vi "FRIC_navX_Get_NextState_ProcessLoop.vi"(11 "I2C Process Loop TypeDef (in)":T1={"State Array"=[enum."INI", enum."Open"], "error"={"status"=FALSE, "code"=0, "source"=""}, "FPGA Cluster"={"Last Valid FPGA Time"=0.0, "Error Count"=0, "Initialized"=FALSE}, "Device Info"={"Interface"={"Protocol"=enum."SERIAL", "Update Rate (4Hz-100Hz)"=4, "navX Open TypeDef"=variant}, "Notify Packet"=refnum, "Loop VI Refnum"=refnum, "Ready to Close Occurrence Refnum"=refnum}, "I2CDevRef"={"DevStatus"={"status"=FALSE, "code"=0, "source"=""}, "Device Address"=0, "Handle"=0, "I2C Bus"=enum."Invalid"}, "Registry"=[], "Command Array"=[214, 32], "Connected?"=FALSE, "navX Device Memory Size"=85, "notification"={"navX Action"=enum."None", "Data"=variant}, "Memory Size Set"=FALSE, "SPIDevRef"={"DevStatus"={"status"=FALSE, "code"=0, "source"=""}, "Handle"=0, "SPI Bus"=enum."SPI On-Board, CS0"}, "navX Serial Open"={"Stream Type"=enum."YRPH", "Serial Port"=enum."Onboard RS-232"}, "SerialPortRef"={"DevStatus"={"status"=FALSE, "code"=0, "source"=""}, "Serial Port Name"=""}, "Serial Read Buffer"="", "Serial Write Buffer"=[], "Device Number"=enum."Dev0", "navX SPI Open"={"SPI Bus"=enum."SPI MXP", "Clock Rate (Hz)"=500000.0}, "Loop dt"=0, "current time"=timestamp(0 s since 1904-01-01), "Loop Time"=0} {"navX Device Memory Size" format="%x"; "Command Array" items=["UNDEFINED"=0, "NAVX_INTEGRATION_CTL_RESET_VEL_X"=1, "NAVX_INTEGRATION_CTL_RESET_VEL_Y"=2, "NAVX_INTEGRATION_CTL_RESET_VEL_Z"=4, "NAVX_INTEGRATION_CTL_RESET_DISP_X"=8, "NAVX_INTEGRATION_CTL_RESET_DISP_Y"=16, "NAVX_INTEGRATION_CTL_RESET_DISP_Z"=32, "NAVX_INTEGRATION_CTL_RESET_YAW"=128]; "I2CDevRef"."Device Address" format="%.0x"; "Device Info"."Interface"."Update Rate (4Hz-100Hz)" min=4 max=60 step=1}) -> (3 "I2C Process Loop TypeDef (out)":T1={"State Array"=[enum."INI", enum."Open"], "error"={"status"=FALSE, "code"=0, "source"=""}, "FPGA Cluster"={"Last Valid FPGA Time"=0.0, "Error Count"=0, "Initialized"=FALSE}, "Device Info"={"Interface"={"Protocol"=enum."SERIAL", "Update Rate (4Hz-100Hz)"=4, "navX Open TypeDef"=variant}, "Notify Packet"=refnum, "Loop VI Refnum"=refnum, "Ready to Close Occurrence Refnum"=refnum}, "I2CDevRef"={"DevStatus"={"status"=FALSE, "code"=0, "source"=""}, "Device Address"=0, "Handle"=0, "I2C Bus"=enum."Invalid"}, "Registry"=[], "Command Array"=[214, 32], "Connected?"=FALSE, "navX Device Memory Size"=85, "notification"={"navX Action"=enum."None", "Data"=variant}, "Memory Size Set"=FALSE, "SPIDevRef"={"DevStatus"={"status"=FALSE, "code"=0, "source"=""}, "Handle"=0, "SPI Bus"=enum."SPI On-Board, CS0"}, "navX Serial Open"={"Stream Type"=enum."YRPH", "Serial Port"=enum."Onboard RS-232"}, "SerialPortRef"={"DevStatus"={"status"=FALSE, "code"=0, "source"=""}, "Serial Port Name"=""}, "Serial Read Buffer"="", "Serial Write Buffer"=[], "Device Number"=enum."Dev0", "navX SPI Open"={"SPI Bus"=enum."SPI MXP", "Clock Rate (Hz)"=500000.0}, "Loop dt"=0, "current time"=timestamp(0 s since 1904-01-01), "Loop Time"=0} {"navX Device Memory Size" format="%x"; "Command Array" items=["UNDEFINED"=0, "NAVX_INTEGRATION_CTL_RESET_VEL_X"=1, "NAVX_INTEGRATION_CTL_RESET_VEL_Y"=2, "NAVX_INTEGRATION_CTL_RESET_VEL_Z"=4, "NAVX_INTEGRATION_CTL_RESET_DISP_X"=8, "NAVX_INTEGRATION_CTL_RESET_DISP_Y"=16, "NAVX_INTEGRATION_CTL_RESET_DISP_Z"=32, "NAVX_INTEGRATION_CTL_RESET_YAW"=128]; "I2CDevRef"."Device Address" format="%.0x"; "Device Info"."Interface"."Update Rate (4Hz-100Hz)" min=4 max=60 step=1}, 5 "Current State":T2)   [LabVIEW 2016]
uses:
  TypeDefs/FRIC_navX_I2C Process Loop TypeDef.ctl
  TypeDefs/FRIC_navX_ProcessingLoopStatesTypeDef_I2C.ctl
  TypeDefs/Z900_navX_DeviceTypeDef.ctl
  TypeDefs/Z900_navX_ProtocolTypeDef.ctl
  TypeDefs/Z900_navX_NotifyPacketTypeDef.ctl
  TypeDefs/Z900_navX_ActionTypeDef.ctl
  <vilib>/Rock Robotics/SystemInterfaces/i2clib/i2c_bus.ctl
  TypeDefs/Z900_navX_IntegrationControlRegisters.ctl
  <vilib>/Rock Robotics/WPI/SPI/WPI_SPIDevRef.ctl
  <vilib>/Rock Robotics/SystemInterfaces/spilib/spi_bus.ctl
  TypeDefs/Z900_navX_SerialStreamTypeDef.ctl
  <vilib>/Rock Robotics/WPI/SerialPort/WPI_SerialPort.ctl
  <vilib>/Rock Robotics/WPI/SerialPort/WPI_SerialPortRef.ctl
  TypeDefs/FRIC_navX_DeviceNumbersTypeDef.ctl
  navX Library v2.lvlib
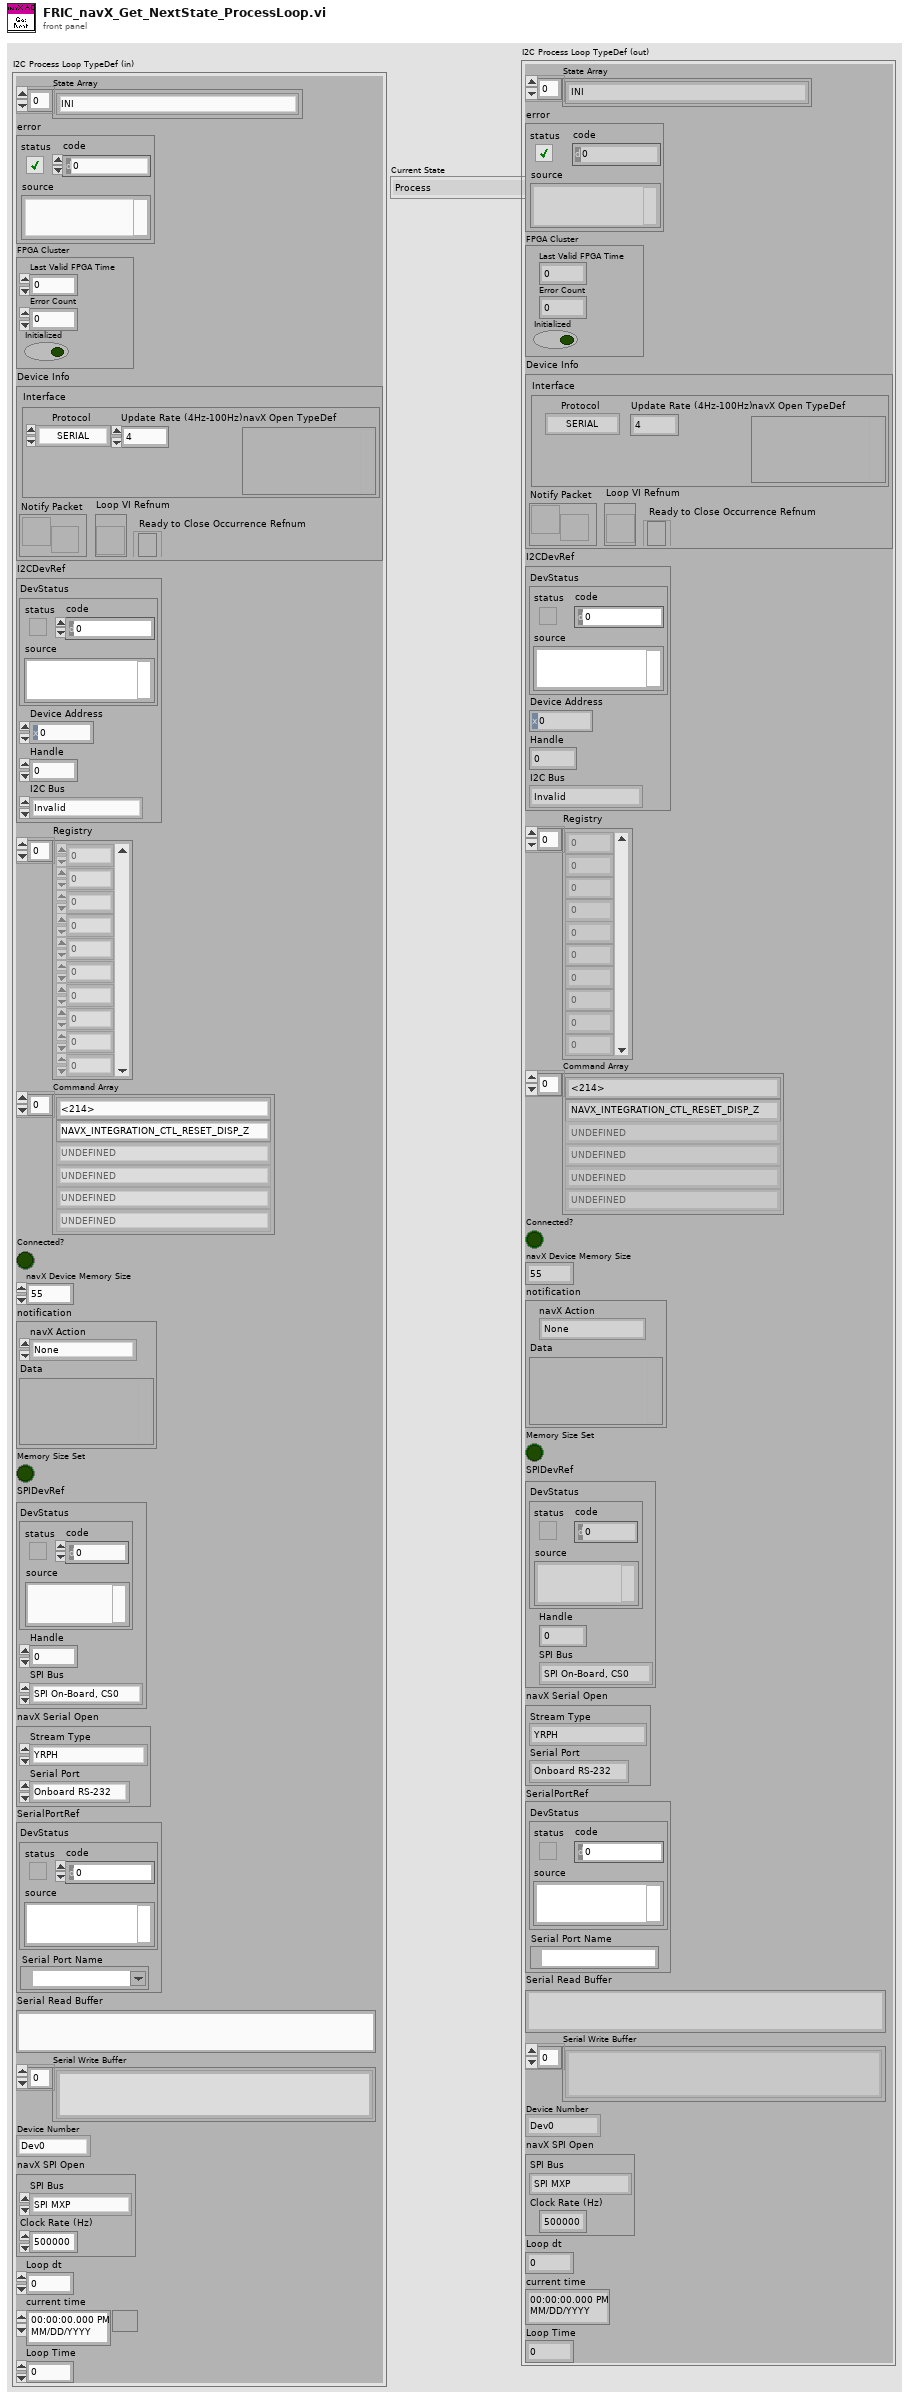
[diagram p1: front panel]
types:
  T1 = typedef "FRIC_navX_I2C Process Loop TypeDef.ctl" = cluster{"State Array":T2[], "error":errorcluster, "FPGA Cluster":cluster{"Last Valid FPGA Time":dbl, "Error Count":i32, "Initialized":bool}, "Device Info":T3, "I2CDevRef":cluster{"DevStatus":errorcluster, "Device Address":u8, "Handle":i32, "I2C Bus":T5}, "Registry":u8[], "Command Array":T6[], "Connected?":bool, "navX Device Memory Size":i32, "notification":T7, "Memory Size Set":bool, "SPIDevRef":T9, "navX Serial Open":cluster{"Stream Type":T11, "Serial Port":T12}, "SerialPortRef":T13, "Serial Read Buffer":string, "Serial Write Buffer":string[], "Device Number":T14, "navX SPI Open":cluster{"SPI Bus":T10, "Clock Rate (Hz)":dbl}, "Loop dt":i64, "current time":timestamp, "Loop Time":i64}
  T2 = typedef "FRIC_navX_ProcessingLoopStatesTypeDef_I2C.ctl" = enum16{"Process", "INI", "Check Packets Valid", "Close", "Flush Serial", "Generate Command", "Last Packet Valid", "Open", "Read", "Reset Serial", "Set Termination Char", "Update AE", "Wait", "Write", "Exit"}
  T3 = typedef "navX Library v2.lvlib/Z900_navX_DeviceTypeDef.ctl" = cluster{"Interface":cluster{"Protocol":T4, "Update Rate (4Hz-100Hz)":u8, "navX Open TypeDef":variant}, "Notify Packet":refnum<notifier>, "Loop VI Refnum":refnum<vi>, "Ready to Close Occurrence Refnum":refnum<k4>}
  T4 = typedef "navX Library v2.lvlib/Z900_navX_ProtocolTypeDef.ctl" = enum16{"SERIAL", "I2C", "SPI"}
  T5 = typedef "i2c_bus.ctl" = enum16{"I2C On-Board", "I2C MXP", "Invalid"}
  T6 = typedef "navX Library v2.lvlib/Z900_navX_IntegrationControlRegisters.ctl" = u8
  T7 = typedef "navX Library v2.lvlib/Z900_navX_NotifyPacketTypeDef.ctl" = cluster{"navX Action":T8, "Data":variant}
  T8 = typedef "navX Library v2.lvlib/Z900_navX_ActionTypeDef.ctl" = enum16{"None", "Halt", "Update Serial Protocol", "Zero-Yaw", "Zero-Displacement", "Zero-Velocity"}
  T9 = typedef "WPI_SPIDevRef.ctl" = cluster{"DevStatus":errorcluster, "Handle":i32, "SPI Bus":T10}
  T10 = typedef "spi_bus.ctl" = enum16{"SPI On-Board, CS0", "SPI On-Board, CS1", "SPI On-Board, CS2", "SPI On-Board, CS3", "SPI MXP", "Invalid"}
  T11 = typedef "navX Library v2.lvlib/Z900_navX_SerialStreamTypeDef.ctl" = enum16{"YRPH", "Quaterinons", "Gyro/Raw", "AHRS", "AHRSAndPositioning"}
  T12 = typedef "WPI_SerialPort.ctl" = enum16{"Onboard RS-232", "MXP TTL", "USB 1", "USB 2"}
  T13 = typedef "WPI_SerialPortRef.ctl" = cluster{"DevStatus":errorcluster, "Serial Port Name":refnum<visa-resource-name>}
  T14 = typedef "FRIC_navX_DeviceNumbersTypeDef.ctl" = enum16{"Dev0", "Dev1", "Dev2", "Dev3"}
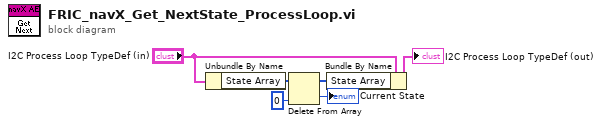
[diagram p0: block diagram]
diagram:
  n1 = Unbundle By Name("I2C Process Loop TypeDef (in)") -> ("State Array"=w5:T2[])
  n2 = Delete From Array(array=w5, index=0) -> (deleted portion=→"Current State":T2, array with subset deleted=w3:T2[])  [unwired: 1 in]
  n3 = Bundle By Name(cluster="I2C Process Loop TypeDef (in)", "State Array"=w3) -> (→"I2C Process Loop TypeDef (out)":T1)
